vi "SaveTempData3.vi"(2 "temp data":dbl[][][](array[numeric]), 3 "Exp_params":T3={"filename"="201612011532", "ExpFilePath"=path "\\\\10.0.0.7\\takada2/DATA/HBT6/data/Test/201612011532.h5", "File Ref list"=[16777216, 33554432], "sweep_dim"=[4, 2], "sweep_list"=[], "readout_list"=["ADC0", "ADC1"], "Sweep instrument bools"=[[0, 0], [0, 0], [0, 0], [0, 0], [0, 0], [0, 0], [0, 0], [0, 0], [0, 0], [0, 0], [0, 0], [0, 0], [0, 0], [0, 0], [0, 0], [0, 0], [0, 0], [0, 0], [0, 0], [0, 0], [0, 0], [0, 0], [0, 0], [0, 0], [0, 0], [0, 0], [0, 0], [0, 0], [0, 0], [0, 0], [0, 0]], "Read out instrument bools"=[[1, 0]], "Experimental bool list"=[FALSE, TRUE], "Initial move"=[{"Name"="None", "kind"=100, "Value"=0.0}], "FPGA Ref"=refnum, "Inst_parameters"={"ConfigFilePath"=path "\\\\10.0.0.7\\takada2/DATA/HBT6/data/Configs/HBT6_ramp_1.h5", "Inst_list"=["ADC", "AWG", "Freq", "Power", "sus", "rus", "rls", "sls", "suq", "suu", "sur", "suc", "sul", "ruq", "ruu", "rur", "ruc", "rul", "rlq", "rlu", "rlr", "rlc", "rll", "slq", "slu", "slr", "slc", "sll", "tu", "t", "tl", "fast_sequence"], "fast_mode"=[1, 1], "Wait_times"=[1, 1, 1, 1], "Inst_array"=[{"Kind"=0, "Strings"=["ADC", "", "V", "ADC0;ADC1", "V;V", "1.0;1.0"], "uint64s"=[10, 2, 250000, 0, 100, 10106, 1000000, 1, 0, 1], "Doubles"=[1.0], "DAQmx take out list"=[]}, {"Kind"=7, "Strings"=["AWG", "10.0.0.4", "", "C:\\Documents and Settings\\Bauerle\\Mes documents\\Bautze\\FPGA-clean_works_1.13.6_batchtest\\Python\\AWG", "dummy", "SAWnstrig_v4.py"], "uint64s"=[2, 0, 0, 3, 0, 0, 0, 0, 0, 0, 0, 0, 0, 0], "Doubles"=[1200000000.0, 1.0, 0.0, 1.0, 0.0, 1.0, 0.0, 1.0, 0.0, 1.0, 0.0, 1.0, 0.0], "DAQmx take out list"=[]}, {"Kind"=6, "Strings"=["Freq", "0:19", "GHz"], "uint64s"=[1, 0, 0, 0, 2, 0, 0, 0], "Doubles"=[2.0, -30.0, 200.0, 100.0, 0.0, 6.000999927520752, 9.000000318337698e-06, 30.0, -145.0], "DAQmx take out list"=[]}, {"Kind"=6, "Strings"=["Power", "0:19", "GHz"], "uint64s"=[1, 0, 1, 0, 2, 0, 0, 0], "Doubles"=[2.0, -30.0, 200.0, 100.0, 0.0, 6.000999927520752, 9.000000318337698e-06, 30.0, -145.0], "DAQmx take out list"=[]}, {"Kind"=4, "Strings"=["sus", "10.0.0.2", "mV"], "uint64s"=[0, 1], "Doubles"=[1.0, -1.0, 1.0, -1.0, 1.0], "DAQmx take out list"=[]}, {"Kind"=4, "Strings"=["rus", "10.0.0.2", "mV"], "uint64s"=[0, 2], "Doubles"=[1.0, -1.0, 1.0, -1.0, 1.0], "DAQmx take out list"=[]}, {"Kind"=4, "Strings"=["rls", "10.0.0.2", "mV"], "uint64s"=[0, 3], "Doubles"=[1.0, -1.0, 1.0, -1.0, 1.0], "DAQmx take out list"=[]}, {"Kind"=4, "Strings"=["sls", "10.0.0.2", "mV"], "uint64s"=[0, 4], "Doubles"=[1.0, -1.0, 1.0, -1.0, 1.0], "DAQmx take out list"=[]}, {"Kind"=4, "Strings"=["suq", "10.0.0.2", "V"], "uint64s"=[0, 5], "Doubles"=[0.30000001192092896, -2.0, 1.0, -1.0, 1.0], "DAQmx take out list"=[]}, {"Kind"=4, "Strings"=["suu", "10.0.0.2", "V"], "uint64s"=[0, 6], "Doubles"=[0.30000001192092896, -2.0, 1.0, -1.0, 1.0], "DAQmx take out list"=[]}, {"Kind"=4, "Strings"=["sur", "10.0.0.2", "V"], "uint64s"=[0, 7], "Doubles"=[0.30000001192092896, -2.0, 1.0, -1.0, 1.0], "DAQmx take out list"=[]}, {"Kind"=4, "Strings"=["suc", "10.0.0.2", "V"], "uint64s"=[1, 0], "Doubles"=[0.30000001192092896, -2.0, 1.0, -1.0, 1.0], "DAQmx take out list"=[]}, {"Kind"=4, "Strings"=["sul", "10.0.0.2", "V"], "uint64s"=[1, 1], "Doubles"=[0.30000001192092896, -2.0, 1.0, -1.0, 1.0], "DAQmx take out list"=[]}, {"Kind"=4, "Strings"=["ruq", "10.0.0.2", "V"], "uint64s"=[1, 2], "Doubles"=[0.30000001192092896, -2.0, 1.0, -1.0, 1.0], "DAQmx take out list"=[]}, {"Kind"=4, "Strings"=["ruu", "10.0.0.2", "V"], "uint64s"=[1, 3], "Doubles"=[0.30000001192092896, -2.0, 1.0, -1.0, 1.0], "DAQmx take out list"=[]}, {"Kind"=4, "Strings"=["rur", "10.0.0.2", "V"], "uint64s"=[1, 5], "Doubles"=[0.30000001192092896, -2.0, 1.0, -1.0, 1.0], "DAQmx take out list"=[]}, {"Kind"=4, "Strings"=["ruc", "10.0.0.2", "V"], "uint64s"=[1, 6], "Doubles"=[0.30000001192092896, -2.0, 1.0, -1.0, 1.0], "DAQmx take out list"=[]}, {"Kind"=4, "Strings"=["rul", "10.0.0.2", "V"], "uint64s"=[1, 7], "Doubles"=[0.30000001192092896, -2.0, 1.0, -1.0, 1.0], "DAQmx take out list"=[]}, {"Kind"=4, "Strings"=["rlq", "10.0.0.2", "V"], "uint64s"=[2, 0], "Doubles"=[0.30000001192092896, -2.0, 1.0, -1.0, 1.0], "DAQmx take out list"=[]}, {"Kind"=4, "Strings"=["rlu", "10.0.0.2", "V"], "uint64s"=[2, 1], "Doubles"=[0.30000001192092896, -2.0, 1.0, -1.0, 1.0], "DAQmx take out list"=[]}, {"Kind"=4, "Strings"=["rlr", "10.0.0.2", "V"], "uint64s"=[2, 2], "Doubles"=[0.30000001192092896, -2.0, 1.0, -1.0, 1.0], "DAQmx take out list"=[]}, {"Kind"=4, "Strings"=["rlc", "10.0.0.2", "V"], "uint64s"=[2, 3], "Doubles"=[0.30000001192092896, -2.0, 1.0, -1.0, 1.0], "DAQmx take out list"=[]}, {"Kind"=4, "Strings"=["rll", "10.0.0.2", "V"], "uint64s"=[2, 4], "Doubles"=[0.30000001192092896, -2.0, 1.0, -1.0, 1.0], "DAQmx take out list"=[]}, {"Kind"=4, "Strings"=["slq", "10.0.0.2", "V"], "uint64s"=[2, 5], "Doubles"=[0.30000001192092896, -2.0, 1.0, -1.0, 1.0], "DAQmx take out list"=[]}, {"Kind"=4, "Strings"=["slu", "10.0.0.2", "V"], "uint64s"=[2, 6], "Doubles"=[0.30000001192092896, -2.0, 1.0, -1.0, 1.0], "DAQmx take out list"=[]}, {"Kind"=4, "Strings"=["slr", "10.0.0.2", "V"], "uint64s"=[2, 7], "Doubles"=[0.30000001192092896, -2.0, 1.0, -1.0, 1.0], "DAQmx take out list"=[]}, {"Kind"=4, "Strings"=["slc", "10.0.0.2", "V"], "uint64s"=[3, 0], "Doubles"=[0.30000001192092896, -2.0, 1.0, -1.0, 1.0], "DAQmx take out list"=[]}, {"Kind"=4, "Strings"=["sll", "10.0.0.2", "V"], "uint64s"=[3, 1], "Doubles"=[0.30000001192092896, -2.0, 1.0, -1.0, 1.0], "DAQmx take out list"=[]}, {"Kind"=4, "Strings"=["tu", "10.0.0.2", "V"], "uint64s"=[3, 2], "Doubles"=[0.30000001192092896, -2.0, 1.0, -1.0, 1.0], "DAQmx take out list"=[]}, {"Kind"=4, "Strings"=["t", "10.0.0.2", "V"], "uint64s"=[3, 3], "Doubles"=[0.30000001192092896, -2.0, 1.0, -1.0, 1.0], "DAQmx take out list"=[]}, {"Kind"=4, "Strings"=["tl", "10.0.0.2", "V"], "uint64s"=[3, 4], "Doubles"=[0.30000001192092896, -2.0, 1.0, -1.0, 1.0], "DAQmx take out list"=[]}, {"Kind"=9, "Strings"=["fast_sequence", "10.0.0.2", "V"], "uint64s"=[6661, 300, 200, 0, 0, 1, 2, 3, 4, 5, 6, 7, 16, 17, 18, 19, 20, 21, 22, 23, 0], "Doubles"=[0.5, -0.5, -1.0, -1.0], "DAQmx take out list"=[]}]}} {"File Ref list" format="%.0x"}, 4 "count":i32) -> (0 "count out":i32)   [LabVIEW 2013]
uses:
  <vilib>/addons/h5labview2/base/hid_t.ctl
  fpga-bitfile-ref.ctl
  <vilib>/addons/h5labview2/file/H5Fmode.ctl
  <vilib>/addons/h5labview2/base/lib_path.vi
  <vilib>/addons/h5labview2/base/H5Equery.vi
  <vilib>/addons/h5labview2/dataset/H5Dwrite.llb/H5Dwrite.xnode
  <vilib>/addons/h5labview2/dataset/H5D.lvlib
  <vilib>/addons/h5labview2/space/H5S.lvlib
  <vilib>/addons/h5labview2/file/H5F.lvlib
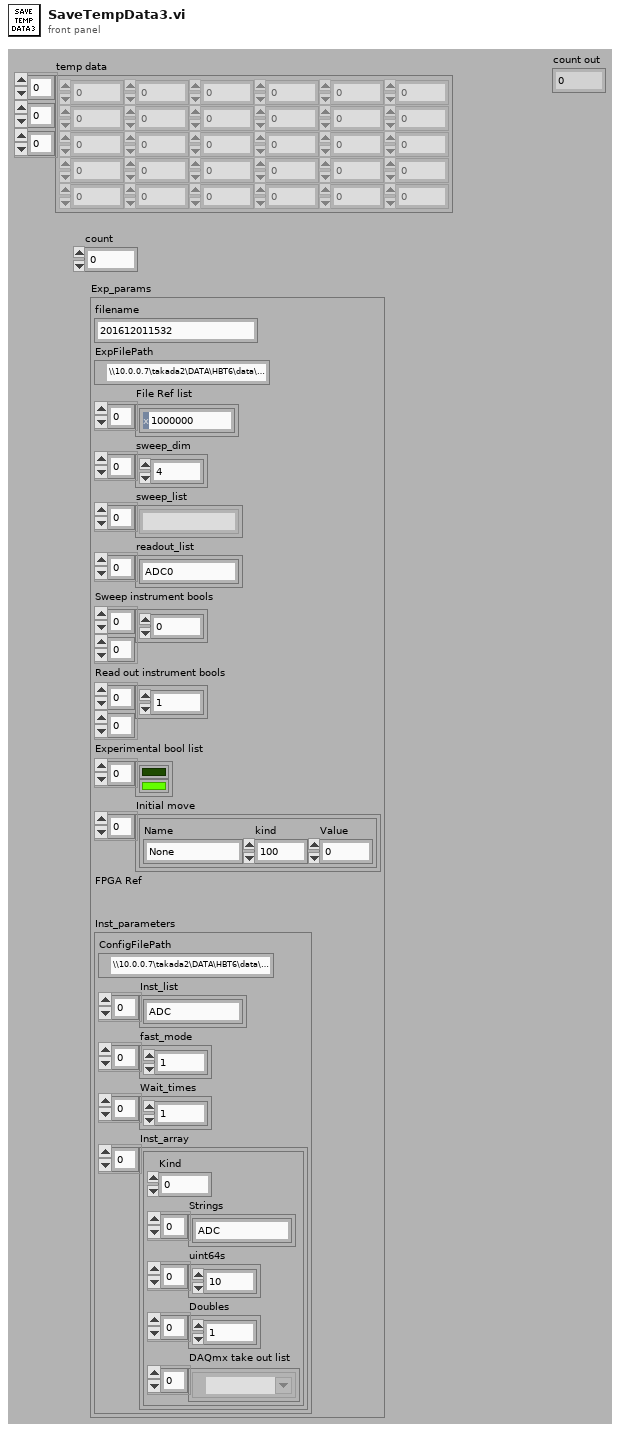
[diagram p1: front panel]
types:
  T1 = typedef "hid_t.ctl" = i32
  T2 = typedef "fpga-bitfile-ref.ctl" = refnum<k20>
  T3 = cluster{"filename":string, "ExpFilePath":path, "File Ref list":T1[], "sweep_dim":u64[], "sweep_list":string[], "readout_list":string[], "Sweep instrument bools":u64[][], "Read out instrument bools":u64[][], "Experimental bool list":bool[], "Initial move":cluster{"Name":string, "kind":u64, "Value":dbl}[], "FPGA Ref":T2, "Inst_parameters":cluster{"ConfigFilePath":path, "Inst_list":string[], "fast_mode":u8[], "Wait_times":u64[], "Inst_array":cluster{"Kind":u16, "Strings":string[], "uint64s":u64[], "Doubles":dbl[], "DAQmx take out list":refnum<k21>[]}[]}}
  T4 = typedef "H5F.lvlib/H5Fmode.ctl" = enum16{"read-only", "read-write", "overwrite", "create new", "open or create"}
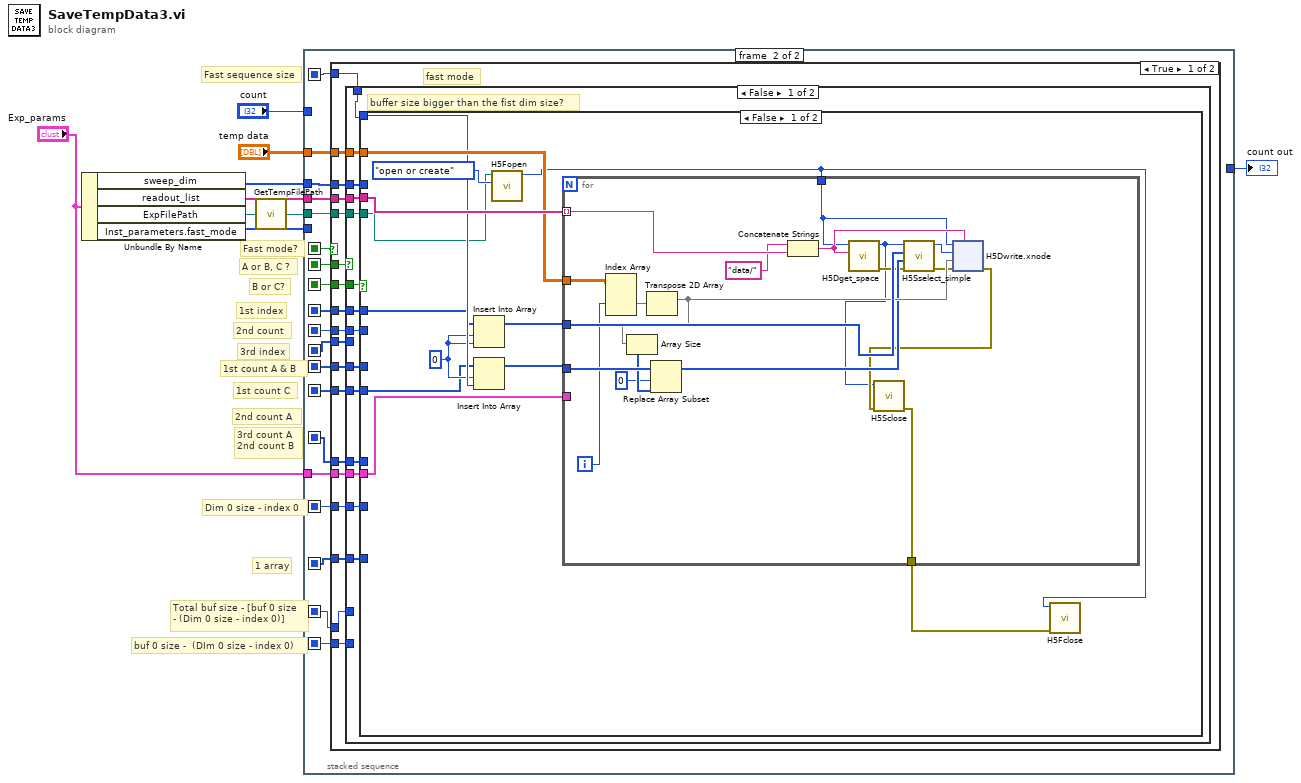
[diagram p0: block diagram]
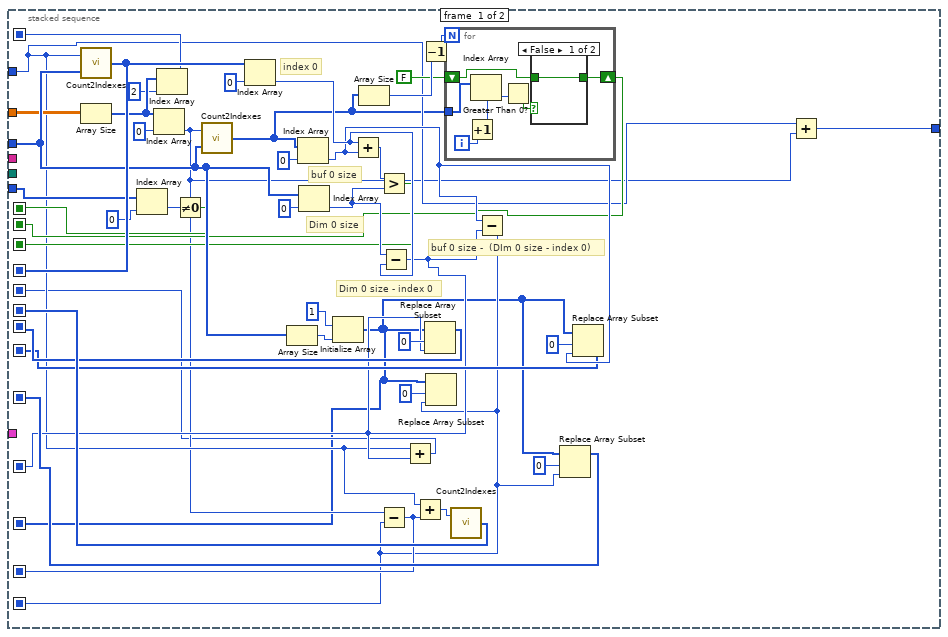
[diagram p2: hidden frame]
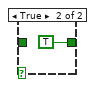
[diagram p3: hidden frame]
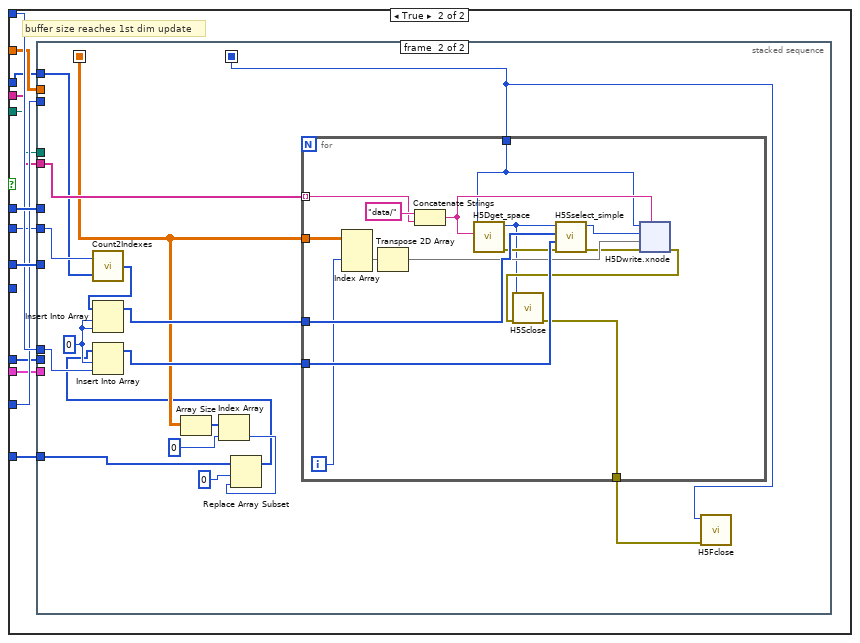
[diagram p4: hidden frame]
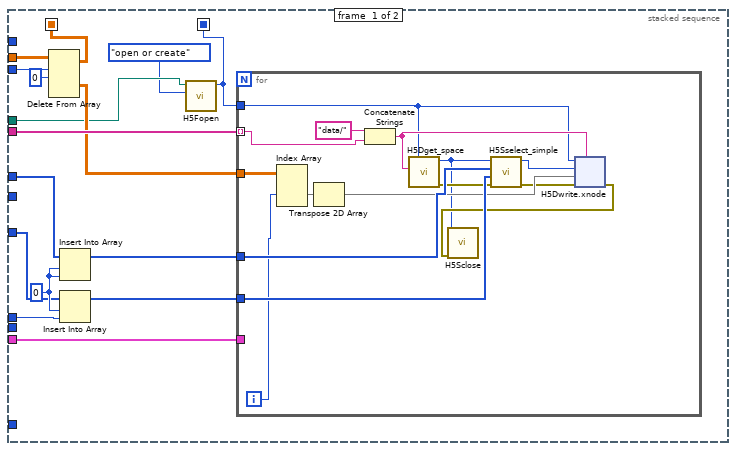
[diagram p5: hidden frame]
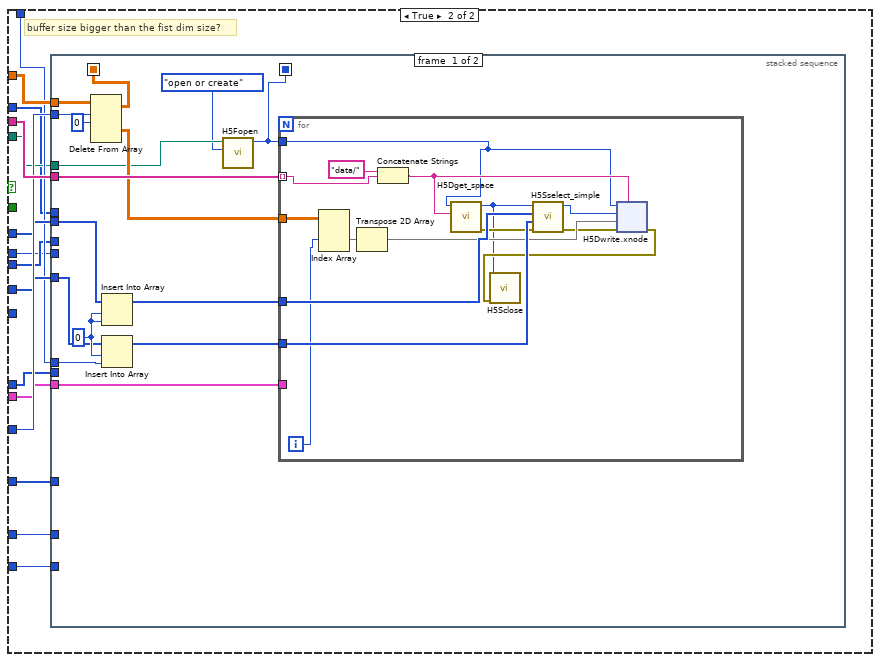
[diagram p6: hidden frame]
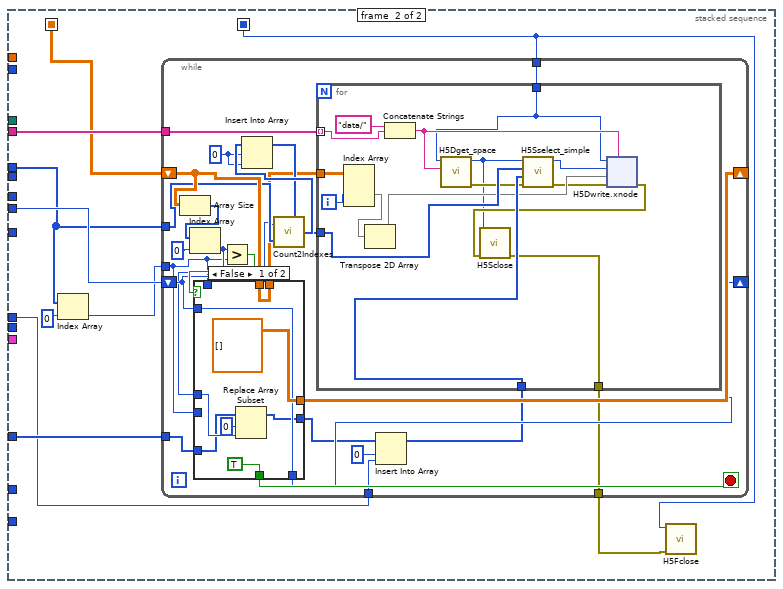
[diagram p7: hidden frame]
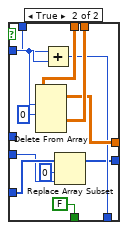
[diagram p8: hidden frame]
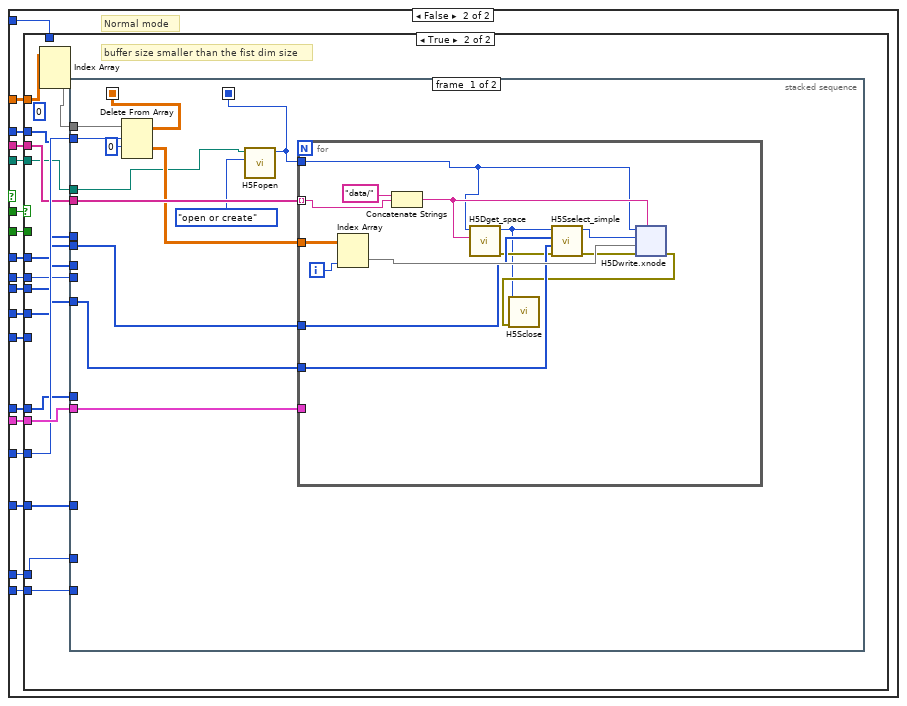
[diagram p9: hidden frame]
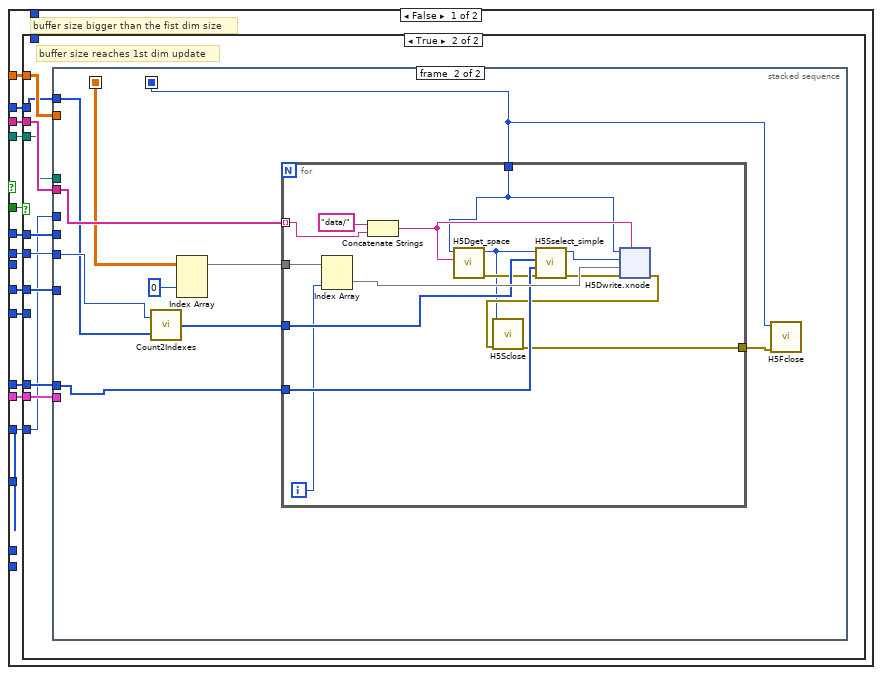
[diagram p10: hidden frame]
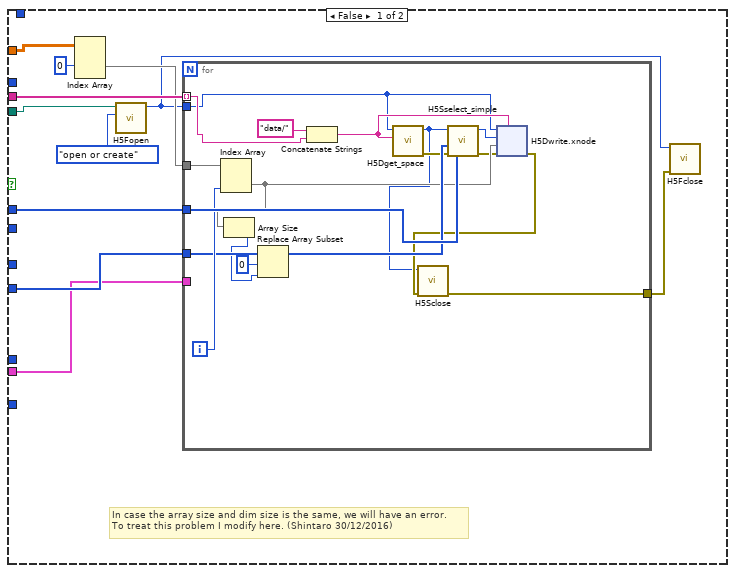
[diagram p11: hidden frame]
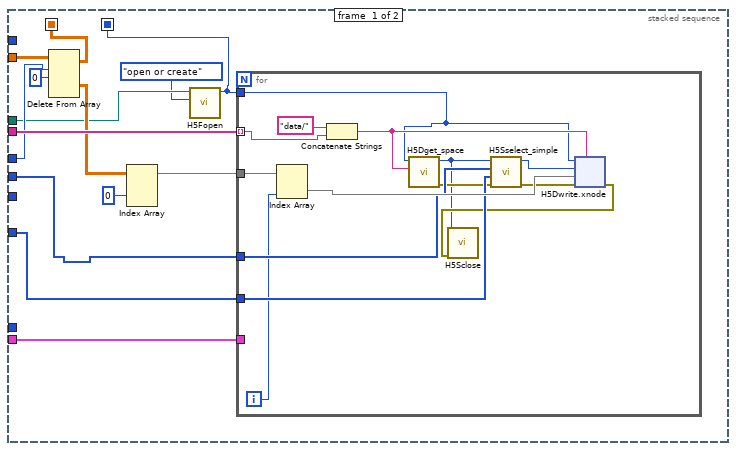
[diagram p12: hidden frame]
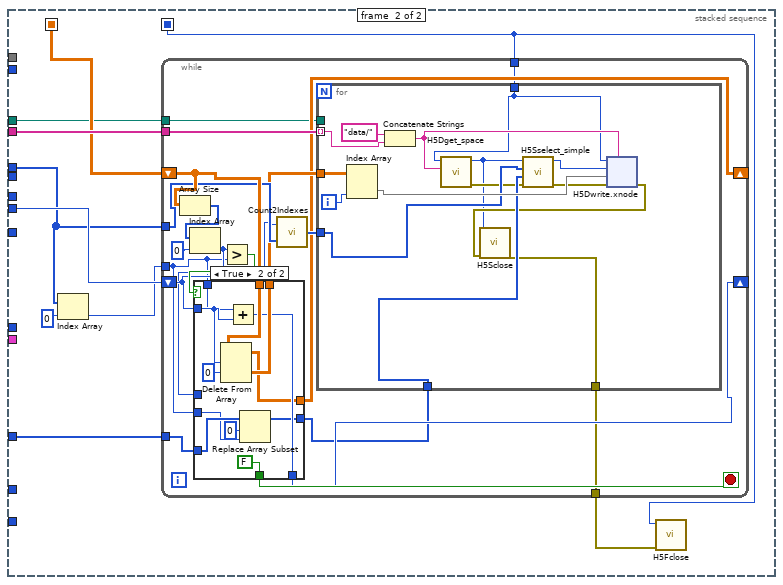
[diagram p13: hidden frame]
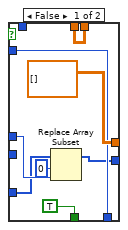
[diagram p14: hidden frame]
diagram:
  # "1 array"
  # "buf 0 size -  (DIm 0 size - index 0)"
  # "Total buf size - [buf 0 size\n- (Dim 0 size - index 0)]"
  # "Dim 0 size - index 0"
  # "Fast sequence size"
  # "B or C?"
  # "A or B, C ?"
  # "Fast mode?"
  # "3rd count A\n2nd count B"
  # "2nd count A"
  # "1st count C"
  # "1st count A & B"
  # "3rd index"
  # "2nd count"
  # "1st index"
  n1 = Unbundle By Name("Exp_params") -> ("sweep_dim"=w7:u64[], "readout_list"=w6:string[], "ExpFilePath"=w2:path, "Inst_parameters.fast_mode"=w5:u8[])
  n2 = call "GetTempFilePath.vi"("ExpFilePath"=w2) -> ("Temp file path"=w1:path)
  n3 = stacked-sequence {
    seq-local: [w48 _] -> [_ w74]
    seq-local: [w11 _] -> [_ w67]
    seq-local: [w36 _] -> [_ w66]
    seq-local: [w35 _] -> [_ w70]
    seq-local: [w32 _] -> [_ w73]
    seq-local: [w29 _] -> [_ w68]
    seq-local: [w22 _] -> [_ w80]
    seq-local: [w26 _] -> [_ w79]
    seq-local: [w27 _] -> [_ w78]
    seq-local: [w19 _] -> [_ w71]
    seq-local: [w18 _] -> [_ w69]
    seq-local: [w14 _] -> [_ w65]
    seq-local: [w13 _] -> [_ w64]
    seq-local: [w10 _] -> [_ w62]
    tunnel: "count" -> [w17 _]
    tunnel: "temp data" -> [w28 w77]
    tunnel: w1 -> [_ w75]
    tunnel: w7 -> [w38 w63]
    tunnel: w6 -> [_ w76]
    tunnel: w5 -> [w25 _]
    tunnel: "Exp_params" -> [_ w72]
    tunnel: [w16 _] -> w3
    frame #0 {
      # "buf 0 size -  (DIm 0 size - index 0)"
      # "Dim 0 size - index 0"
      # "Dim 0 size"
      # "buf 0 size"
      # "index 0"
      n4 = call "Count2Indexes.vi"("sweep_dim"=w38, "Count"=w17) -> ("Indexes"=w48:u64[])
      n5 = Array Size(array=w28) -> (size(s)=w21:i32[])
      n6 = Index Array(array=w25, index=0) -> (element=w23:u8)
      n7 = Index Array(array=w21, index=0) -> (element=w15:i32)
      n8 = Index Array(array=w21, index=2) -> (element=w19:i32)
      n9 = Not Equal To 0?(x=w23) -> (x != 0?=w22:bool)
      n10 = call "Count2Indexes.vi"("sweep_dim"=w38, "Count"=w15) -> ("Indexes"=w12:u64[])
      n11 = Index Array(array=w48, index=0) -> (element=w43:u64)
      n12 = Array Size(array=w38) -> (size(s)=w42:i32)
      n13 = Index Array(array=w12, index=0) -> (element=w33:u64)
      n14 = Index Array(array=w38, index=0) -> (element=w31:u64)
      n15 = Initialize Array(1, w42) -> (w10:i32[])
      n16 = Add(x=w43, y=w33) -> (x+y=w47:u64)
      n17 = Array Size(array=w12) -> (size(s)=w46:i32)
      n18 = Greater?(x=w47, y=w31) -> (0:w27:bool)
      n19 = Subtract(x=w31, y=w43) -> (x-y=w18:u64)
      n20 = Add(x=w17, y=w18) -> (x+y=w11:u64)
      n21 = Decrement(x=w46) -> (x-1=w45:i32)
      n22 = Replace Array Subset(array=w10, new element=w18, index=0) -> (w35:i32[])
      n23 = for {
        N: w45 -> [_]
        tunnel: w12 -> [w59]
        shift-right: [w53] -> w26
        shift-left: FALSE -> [w54]
        i -> [w58]
        n24 = Increment(x=w58) -> (x+1=w57:i32)
        n25 = Index Array(array=w59, index=w57) -> (element=w56:u64)
        n26 = Greater Than 0?(x=w56) -> (x > 0?=w55:bool)
        n27 = case shown="False" w55 {
          tunnel: w54 -> [w60 _]
          tunnel: [w60 TRUE] -> w53
          frame False {
          }
          frame True {
          }
        }
      }
      n28 = Subtract(x=w33, y=w18) -> (x-y=w13:u64)
      n29 = Subtract(x=w15, y=w13) -> (x-y=w14:u64)
      n30 = Add(x=w17, y=w14) -> (x+y=w37:u64)
      n31 = Replace Array Subset(array=w10, new element=w13, index=0) -> ()  [unwired: 1 out]
      n32 = call "Count2Indexes.vi"("Count"=w37) -> ("Indexes"=w36:u64[])  [unwired: 1 in]
      n33 = Replace Array Subset(array=w10, new element=w13, index=0) -> (w29:i32[])
      n34 = Replace Array Subset(array=w10, new element=w33, index=0) -> (w32:i32[])
      n35 = Add(x=w17, y=w15) -> (x+y=w16:i32)
    }
    frame #1 {
      n36 = case shown="True" w80 {
        tunnel: w79 -> [w98 w443]
        tunnel: w78 -> [w97 w442]
        tunnel: w77 -> [w95 w441]
        tunnel: w76 -> [w96 w440]
        tunnel: w75 -> [w94 w439]
        tunnel: w74 -> [w91 w438]
        tunnel: w73 -> [w90 w437]
        tunnel: w72 -> [w93 w436]
        tunnel: w71 -> [w92 w434]
        tunnel: w70 -> [w89 w435]
        tunnel: w69 -> [w88 w431]
        tunnel: w68 -> [w87 w433]
        tunnel: w67 -> [w86 w432]
        tunnel: w66 -> [w85 w426]
        tunnel: w65 -> [w84 w430]
        tunnel: w64 -> [w83 w429]
        tunnel: w63 -> [w82 w428]
        tunnel: w62 -> [w81 w427]
        frame True {
          # "fast mode"
          n37 = case shown="False" w98 {
            tunnel: w97 -> [w112 _]
            tunnel: w96 -> [w111 w288]
            tunnel: w95 -> [w110 w289]
            tunnel: w94 -> [w109 w280]
            tunnel: w93 -> [w108 w283]
            tunnel: w92 -> [w107 w284]
            tunnel: w91 -> [w106 w286]
            tunnel: w90 -> [w105 _]
            tunnel: w89 -> [w104 w285]
            tunnel: w88 -> [w103 w287]
            tunnel: w87 -> [w102 w281]
            tunnel: w86 -> [w101 w279]
            tunnel: w85 -> [_ w282]
            tunnel: w84 -> [_ w278]
            tunnel: w83 -> [_ w277]
            tunnel: w82 -> [w100 w276]
            tunnel: w81 -> [w99 w275]
            frame False {
              # "buffer size bigger than the fist dim size?"
              n38 = case shown="False" w112 {
                tunnel: w111 -> [w125 w169]
                tunnel: w110 -> [w124 w171]
                tunnel: w109 -> [w115 w168]
                tunnel: w108 -> [w123 w167]
                tunnel: w107 -> [w122 w172]
                tunnel: w106 -> [w120 w173]
                tunnel: w105 -> [w119 _]
                tunnel: w104 -> [_ w174]
                tunnel: w103 -> [_ w170]
                tunnel: w102 -> [_ w166]
                tunnel: w101 -> [_ w165]
                tunnel: w100 -> [_ w164]
                tunnel: w99 -> [_ w163]
                frame False {
                  w121 = 0
                  n39 = Insert Into Array(array=w120, index=w121, new element=w121) -> (w118:u64[])
                  n40 = Insert Into Array(array=w119, index=w121, new element=w122) -> (w117:i32[])
                  n41 = call <vilib>:"H5Fopen.vi"("mode (read-only)"=H5Fmode."open or create" ("mode"), "path"=w115) -> ("ref out"=w113:T1)  [unwired: 8 in, 1 out]
                  n42 = for {
                    tunnel: w118 -> [w144]
                    tunnel: w125 -> [w143] mode=indexing
                    tunnel: w124 -> [w142]
                    tunnel: w117 -> [w140]
                    tunnel: w123 -> [_]
                    tunnel: w113 -> [w127]
                    tunnel: [w126] -> w114
                    i -> [w139]
                    n43 = Index Array(array=w142, index (dim 1)=w139) -> (element=w141:dbl[][])  [unwired: 2 in]
                    n44 = Transpose 2D Array(2D array=w141) -> (transposed array=w138:dbl[][])
                    n45 = Array Size(array=w138) -> (size(s)=w136:i32[])
                    n46 = Replace Array Subset(array=w140, new element=w136, index=0) -> (w137:i32[])
                    n47 = Concatenate Strings("data/", w143) -> (w129:string)
                    n48 = call <vilib>:"H5Dget_space.vi"("obj (.)"=w129, "ref in"=w127) -> ("error out"=w134:errorcluster, "space out"=w130:T1)  [unwired: 8 in]
                    n49 = call <vilib>:"H5Sselect_simple.vi"("error in (no error)"=w134, "count"=w137, "start"=w144, "space in"=w130) -> ("error out"=w133:errorcluster, "space out"=w132:T1)  [unwired: 6 in]
                    n50 = xnode "H5Dwrite.xnode"("dataset name"=w129, "error in (no error)"=w133, "data"=w138, "file space"=w132, "ref in"=w127) -> ("error out"=w131:errorcluster)  [unwired: 2 in, 2 out]
                    n51 = call <vilib>:"H5Sclose.vi"("error in (no error)"=w131, "space in"=w130) -> ("error out"=w126:errorcluster)  [unwired: 9 in]
                  }
                  n52 = call <vilib>:"H5Fclose.vi"("error in (no error)"=w114, "ref"=w113) -> ()  [unwired: 9 in, 1 out]
                }
                frame True {
                  # "buffer size reaches 1st dim update"
                  n53 = stacked-sequence {
                    seq-local: [w183 _] -> [_ w232]
                    seq-local: [w175 _] -> [_ w224]
                    tunnel: w174 -> [w189 _]
                    tunnel: w173 -> [w188 _]
                    tunnel: w172 -> [w187 w238]
                    tunnel: w171 -> [w186 _]
                    tunnel: w170 -> [w185 _]
                    tunnel: w169 -> [w182 w240]
                    tunnel: w168 -> [w177 _]
                    tunnel: w167 -> [w178 _]
                    tunnel: w166 -> [_ _]
                    tunnel: w165 -> [_ w235]
                    tunnel: w164 -> [_ w233]
                    tunnel: w163 -> [_ w229]
                    frame #0 {
                      w190 = 0
                      n54 = Delete From Array(array=w186, length=w185, index (dim 0)=0) -> (deleted portion=w181:dbl[][][], array with subset deleted=w183:dbl[][][])  [unwired: 2 in]
                      n55 = Insert Into Array(array=w188, index=w190, new element=w190) -> (w179:u64[])
                      n56 = Insert Into Array(array=w189, index=w190, new element=w187) -> (w180:i32[])
                      n57 = call <vilib>:"H5Fopen.vi"("mode (read-only)"=H5Fmode."open or create" ("mode"), "path"=w177) -> ("ref out"=w175:T1)  [unwired: 8 in, 1 out]
                      n58 = for {
                        tunnel: w182 -> [w193] mode=indexing
                        tunnel: w181 -> [w205]
                        tunnel: w180 -> [w203]
                        tunnel: w179 -> [w202]
                        tunnel: w178 -> [_]
                        tunnel: w175 -> [w191]
                        i -> [w201]
                        n59 = Index Array(array=w205, index (dim 1)=w201) -> (element=w204:dbl[][])  [unwired: 2 in]
                        n60 = Transpose 2D Array(2D array=w204) -> (transposed array=w200:dbl[][])
                        n61 = Concatenate Strings("data/", w193) -> (w192:string)
                        n62 = call <vilib>:"H5Dget_space.vi"("obj (.)"=w192, "ref in"=w191) -> ("error out"=w199:errorcluster, "space out"=w195:T1)  [unwired: 8 in]
                        n63 = call <vilib>:"H5Sselect_simple.vi"("error in (no error)"=w199, "count"=w203, "start"=w202, "space in"=w195) -> ("error out"=w198:errorcluster, "space out"=w197:T1)  [unwired: 6 in]
                        n64 = xnode "H5Dwrite.xnode"("dataset name"=w192, "error in (no error)"=w198, "data"=w200, "file space"=w197, "ref in"=w191) -> ("error out"=w196:errorcluster)  [unwired: 2 in, 2 out]
                        n65 = call <vilib>:"H5Sclose.vi"("error in (no error)"=w196, "space in"=w195) -> ()  [unwired: 9 in, 1 out]
                      }
                    }
                    frame #1 {
                      w239 = 0
                      n66 = call "Count2Indexes.vi"("sweep_dim"=w233, "Count"=w235) -> ("Indexes"=w234:u64[])
                      n67 = Insert Into Array(array=w234, index=w239, new element=w239) -> (w236:u64[])
                      n68 = Array Size(array=w232) -> (size(s)=w231:i32[])
                      n69 = Index Array(array=w231, index=0) -> (element=w228:i32)
                      n70 = Replace Array Subset(array=w229, new element=w228, index=0) -> (w226:i32[])
                      n71 = Insert Into Array(array=w226, index=w239, new element=w238) -> (w237:i32[])
                      n72 = for {
                        tunnel: w240 -> [w244] mode=indexing
                        tunnel: w232 -> [w256]
                        tunnel: w237 -> [w254]
                        tunnel: w236 -> [w253]
                        tunnel: w224 -> [w242]
                        tunnel: [w241] -> w225
                        i -> [w252]
                        n73 = Index Array(array=w256, index (dim 1)=w252) -> (element=w255:dbl[][])  [unwired: 2 in]
                        n74 = Transpose 2D Array(2D array=w255) -> (transposed array=w251:dbl[][])
                        n75 = Concatenate Strings("data/", w244) -> (w243:string)
                        n76 = call <vilib>:"H5Dget_space.vi"("obj (.)"=w243, "ref in"=w242) -> ("error out"=w250:errorcluster, "space out"=w246:T1)  [unwired: 8 in]
                        n77 = call <vilib>:"H5Sselect_simple.vi"("error in (no error)"=w250, "count"=w254, "start"=w253, "space in"=w246) -> ("error out"=w249:errorcluster, "space out"=w248:T1)  [unwired: 6 in]
                        n78 = xnode "H5Dwrite.xnode"("dataset name"=w243, "error in (no error)"=w249, "data"=w251, "file space"=w248, "ref in"=w242) -> ("error out"=w247:errorcluster)  [unwired: 2 in, 2 out]
                        n79 = call <vilib>:"H5Sclose.vi"("error in (no error)"=w247, "space in"=w246) -> ("error out"=w241:errorcluster)  [unwired: 9 in]
                      }
                      n80 = call <vilib>:"H5Fclose.vi"("error in (no error)"=w225, "ref"=w224) -> ()  [unwired: 9 in, 1 out]
                    }
                  }
                }
              }
            }
            frame True {
              # "buffer size bigger than the fist dim size?"
              n81 = stacked-sequence {
                seq-local: [w298 _] -> [_ w341]
                seq-local: [w290 _] -> [_ w339]
                tunnel: w285 -> [w304 _]
                tunnel: w286 -> [w303 _]
                tunnel: w284 -> [w302 w342]
                tunnel: w289 -> [w301 _]
                tunnel: w287 -> [w300 _]
                tunnel: w288 -> [w297 w348]
                tunnel: w280 -> [w292 _]
                tunnel: w283 -> [w294 _]
                tunnel: w281 -> [_ _]
                tunnel: w282 -> [_ _]
                tunnel: w279 -> [_ w347]
                tunnel: w278 -> [_ _]
                tunnel: w277 -> [_ _]
                tunnel: w276 -> [_ w346]
                tunnel: w275 -> [_ w343]
                frame #0 {
                  w305 = 0
                  n82 = Delete From Array(array=w301, length=w300, index (dim 0)=0) -> (deleted portion=w296:dbl[][][], array with subset deleted=w298:dbl[][][])  [unwired: 2 in]
                  n83 = Insert Into Array(array=w303, index=w305, new element=w305) -> (w295:u64[])
                  n84 = Insert Into Array(array=w304, index=w305, new element=w302) -> (w293:i32[])
                  n85 = call <vilib>:"H5Fopen.vi"("mode (read-only)"=H5Fmode."open or create" ("mode"), "path"=w292) -> ("ref out"=w290:T1)  [unwired: 8 in, 1 out]
                  n86 = for {
                    tunnel: w297 -> [w308] mode=indexing
                    tunnel: w296 -> [w320]
                    tunnel: w293 -> [w318]
                    tunnel: w295 -> [w317]
                    tunnel: w294 -> [_]
                    tunnel: w290 -> [w306]
                    i -> [w316]
                    n87 = Index Array(array=w320, index (dim 1)=w316) -> (element=w319:dbl[][])  [unwired: 2 in]
                    n88 = Transpose 2D Array(2D array=w319) -> (transposed array=w315:dbl[][])
                    n89 = Concatenate Strings("data/", w308) -> (w307:string)
                    n90 = call <vilib>:"H5Dget_space.vi"("obj (.)"=w307, "ref in"=w306) -> ("error out"=w314:errorcluster, "space out"=w310:T1)  [unwired: 8 in]
                    n91 = call <vilib>:"H5Sselect_simple.vi"("error in (no error)"=w314, "count"=w318, "start"=w317, "space in"=w310) -> ("error out"=w313:errorcluster, "space out"=w312:T1)  [unwired: 6 in]
                    n92 = xnode "H5Dwrite.xnode"("dataset name"=w307, "error in (no error)"=w313, "data"=w315, "file space"=w312, "ref in"=w306) -> ("error out"=w311:errorcluster)  [unwired: 2 in, 2 out]
                    n93 = call <vilib>:"H5Sclose.vi"("error in (no error)"=w311, "space in"=w310) -> ()  [unwired: 9 in, 1 out]
                  }
                }
                frame #1 {
                  n94 = Index Array(array=w346, index=0) -> (element=w344:u64)
                  n95 = while {
                    tunnel: w348 -> [w371]
                    shift-right: [w365] -> _
                    shift-left: w341 -> [w367]
                    tunnel: w346 -> [w363]
                    shift-right: [w364] -> _
                    shift-left: w347 -> [w362]
                    tunnel: w344 -> [w356]
                    tunnel: w343 -> [w355]
                    tunnel: w342 -> [w352]
                    tunnel: w339 -> [w350]
                    tunnel: [w349] -> w340
                    stop <- w366 stop-if-true
                    w360 = 0
                    n96 = Array Size(array=w367) -> (size(s)=w370:i32[])
                    n97 = Index Array(array=w370, index=0) -> (element=w357:i32)
                    n98 = Greater?(x=w357, y=w356) -> (0:w368:bool)
                    n99 = case shown="False" w368 {
                      tunnel: w362 -> [w376 w391]
                      tunnel: w356 -> [_ w387]
                      tunnel: w367 -> [w378 w390]
                      tunnel: [w378 w389] -> w358
                      tunnel: [TRUE FALSE] -> w366
                      tunnel: [dbl[][][] [] w385] -> w365
                      tunnel: [w376 w384] -> w364
                      tunnel: w357 -> [w373 _]
                      tunnel: w356 -> [_ w382]
                      tunnel: w355 -> [w372 w383]
                      tunnel: [w374 w380] -> w354
                      frame False {
                        n100 = Replace Array Subset(array=w372, new element=w373, index=0) -> (w374:i32[])
                      }
                      frame True {
                        n101 = Delete From Array(array=w390, length=w387, index (dim 0)=0) -> (deleted portion=w389:dbl[][][], array with subset deleted=w385:dbl[][][])  [unwired: 2 in]
                        n102 = Add(x=w387, y=w391) -> (x+y=w384:u64)
                        n103 = Replace Array Subset(array=w383, new element=w382, index=0) -> (w380:i32[])
                      }
                    }
                    n104 = call "Count2Indexes.vi"("sweep_dim"=w363, "Count"=w362) -> ("Indexes"=w361:u64[])
                    n105 = Insert Into Array(array=w361, index=w360, new element=w360) -> (w359:u64[])
                    n106 = Insert Into Array(array=w354, index=0, new element=w352) -> (w351:i32[])
                    n107 = for {
                      tunnel: w371 -> [w395] mode=indexing
                      tunnel: w358 -> [w407]
                      tunnel: w359 -> [w406]
                      tunnel: w351 -> [w405]
                      tunnel: w350 -> [w393]
                      tunnel: [w392] -> w349
                      i -> [w404]
                      n108 = Index Array(array=w407, index (dim 1)=w404) -> (element=w403:dbl[][])  [unwired: 2 in]
                      n109 = Transpose 2D Array(2D array=w403) -> (transposed array=w402:dbl[][])
                      n110 = Concatenate Strings("data/", w395) -> (w394:string)
                      n111 = call <vilib>:"H5Dget_space.vi"("obj (.)"=w394, "ref in"=w393) -> ("error out"=w401:errorcluster, "space out"=w397:T1)  [unwired: 8 in]
                      n112 = call <vilib>:"H5Sselect_simple.vi"("error in (no error)"=w401, "count"=w405, "start"=w406, "space in"=w397) -> ("error out"=w400:errorcluster, "space out"=w399:T1)  [unwired: 6 in]
                      n113 = xnode "H5Dwrite.xnode"("dataset name"=w394, "error in (no error)"=w400, "data"=w402, "file space"=w399, "ref in"=w393) -> ("error out"=w398:errorcluster)  [unwired: 2 in, 2 out]
                      n114 = call <vilib>:"H5Sclose.vi"("error in (no error)"=w398, "space in"=w397) -> ("error out"=w392:errorcluster)  [unwired: 9 in]
                    }
                  }
                  n115 = call <vilib>:"H5Fclose.vi"("error in (no error)"=w340, "ref"=w339) -> ()  [unwired: 9 in, 1 out]
                }
              }
            }
          }
        }
        frame False {
          # "Normal mode"
          n116 = case shown="True" w443 {
            tunnel: w442 -> [w456 _]
            tunnel: w441 -> [w455 w605]
            tunnel: w440 -> [w454 w616]
            tunnel: w439 -> [w453 w615]
            tunnel: w438 -> [w452 w614]
            tunnel: w437 -> [w451 _]
            tunnel: w436 -> [w450 w618]
            tunnel: w435 -> [w449 w613]
            tunnel: w434 -> [w448 _]
            tunnel: w433 -> [w447 w606]
            tunnel: w432 -> [w446 w609]
            tunnel: w431 -> [w445 w617]
            tunnel: w430 -> [_ w612]
            tunnel: w429 -> [_ w611]
            tunnel: w428 -> [w444 w610]
            tunnel: w427 -> [_ w608]
            tunnel: w426 -> [_ w607]
            frame False {
              # "buffer size bigger than the fist dim size"
              n117 = case shown="True" w456 {
                tunnel: w455 -> [w465 w513]
                tunnel: w454 -> [w466 w512]
                tunnel: w453 -> [w460 w511]
                tunnel: w452 -> [w467 w510]
                tunnel: w451 -> [w462 _]
                tunnel: w450 -> [w461 w508]
                tunnel: w449 -> [_ w509]
                tunnel: w448 -> [_ _]
                tunnel: w447 -> [_ w507]
                tunnel: w446 -> [_ w506]
                tunnel: w445 -> [_ w505]
                tunnel: w444 -> [_ w504]
                frame False {
                  # "In case the array size and dim size is the same, we will have an error.\nTo treat this problem I modify here. (Shintaro 30/12/2016)"
                  n118 = Index Array(array=w465, index (dim 1)=0) -> (element=w463:dbl[][])  [unwired: 2 in]
                  n119 = call <vilib>:"H5Fopen.vi"("mode (read-only)"=H5Fmode."open or create" ("mode"), "path"=w460) -> ("ref out"=w457:T1)  [unwired: 8 in, 1 out]
                  n120 = for {
                    tunnel: w467 -> [w485]
                    tunnel: w466 -> [w470] mode=indexing
                    tunnel: w463 -> [w484]
                    tunnel: w462 -> [w482]
                    tunnel: w461 -> [_]
                    tunnel: w457 -> [w469]
                    tunnel: [w468] -> w458
                    i -> [w483]
                    n121 = Index Array(array=w484, index (col)=w483) -> (element=w479:dbl[])  [unwired: 1 in]
                    n122 = Array Size(array=w479) -> (size(s)=w478:i32)
                    n123 = Replace Array Subset(array=w482, new element=w478, index=0) -> (w481:i32[])
                    n124 = Concatenate Strings("data/", w470) -> (w471:string)
                    n125 = call <vilib>:"H5Dget_space.vi"("obj (.)"=w471, "ref in"=w469) -> ("error out"=w477:errorcluster, "space out"=w473:T1)  [unwired: 8 in]
                    n126 = call <vilib>:"H5Sselect_simple.vi"("error in (no error)"=w477, "count"=w481, "start"=w485, "space in"=w473) -> ("error out"=w476:errorcluster, "space out"=w475:T1)  [unwired: 6 in]
                    n127 = xnode "H5Dwrite.xnode"("dataset name"=w471, "error in (no error)"=w476, "data"=w479, "file space"=w475, "ref in"=w469) -> ("error out"=w474:errorcluster)  [unwired: 2 in, 2 out]
                    n128 = call <vilib>:"H5Sclose.vi"("error in (no error)"=w474, "space in"=w473) -> ("error out"=w468:errorcluster)  [unwired: 9 in]
                  }
                  n129 = call <vilib>:"H5Fclose.vi"("error in (no error)"=w458, "ref"=w457) -> ()  [unwired: 9 in, 1 out]
                }
                frame True {
                  # "buffer size reaches 1st dim update"
                  n130 = stacked-sequence {
                    seq-local: [w525 _] -> [_ w568]
                    seq-local: [w514 _] -> [_ w560]
                    tunnel: w509 -> [w517 _]
                    tunnel: w510 -> [w518 _]
                    tunnel: w513 -> [w527 _]
                    tunnel: w512 -> [w524 w569]
                    tunnel: w511 -> [w516 _]
                    tunnel: w508 -> [w522 _]
                    tunnel: w507 -> [_ w567]
                    tunnel: w506 -> [_ w563]
                    tunnel: w505 -> [w521 _]
                    tunnel: w504 -> [_ w562]
                    frame #0 {
                      n131 = Delete From Array(array=w527, length=w521, index (dim 0)=0) -> (deleted portion=w523:dbl[][][], array with subset deleted=w525:dbl[][][])  [unwired: 2 in]
                      n132 = Index Array(array=w523, index (dim 1)=0) -> (element=w520:dbl[][])  [unwired: 2 in]
                      n133 = call <vilib>:"H5Fopen.vi"("mode (read-only)"=H5Fmode."open or create" ("mode"), "path"=w516) -> ("ref out"=w514:T1)  [unwired: 8 in, 1 out]
                      n134 = for {
                        tunnel: w524 -> [w529] mode=indexing
                        tunnel: w520 -> [w541]
                        tunnel: w517 -> [w539]
                        tunnel: w518 -> [w538]
                        tunnel: w522 -> [_]
                        tunnel: w514 -> [w528]
                        i -> [w537]
                        n135 = Index Array(array=w541, index (col)=w537) -> (element=w540:dbl[])  [unwired: 1 in]
                        n136 = Concatenate Strings("data/", w529) -> (w530:string)
                        n137 = call <vilib>:"H5Dget_space.vi"("obj (.)"=w530, "ref in"=w528) -> ("error out"=w536:errorcluster, "space out"=w532:T1)  [unwired: 8 in]
                        n138 = call <vilib>:"H5Sselect_simple.vi"("error in (no error)"=w536, "count"=w539, "start"=w538, "space in"=w532) -> ("error out"=w535:errorcluster, "space out"=w534:T1)  [unwired: 6 in]
                        n139 = xnode "H5Dwrite.xnode"("dataset name"=w530, "error in (no error)"=w535, "data"=w540, "file space"=w534, "ref in"=w528) -> ("error out"=w533:errorcluster)  [unwired: 2 in, 2 out]
                        n140 = call <vilib>:"H5Sclose.vi"("error in (no error)"=w533, "space in"=w532) -> ()  [unwired: 9 in, 1 out]
                      }
                    }
                    frame #1 {
                      n141 = call "Count2Indexes.vi"("sweep_dim"=w562, "Count"=w563) -> ("Indexes"=w564:u64[])
                      n142 = Index Array(array=w568, index (dim 1)=0) -> (element=w566:dbl[][])  [unwired: 2 in]
                      n143 = for {
                        tunnel: w569 -> [w574] mode=indexing
                        tunnel: w566 -> [w584]
                        tunnel: w567 -> [w582]
                        tunnel: w564 -> [w581]
                        tunnel: w560 -> [w571]
                        tunnel: [w570] -> w561
                        i -> [w580]
                        n144 = Index Array(array=w584, index (col)=w580) -> (element=w583:dbl[])  [unwired: 1 in]
                        n145 = Concatenate Strings("data/", w574) -> (w573:string)
                        n146 = call <vilib>:"H5Dget_space.vi"("obj (.)"=w573, "ref in"=w571) -> ("error out"=w579:errorcluster, "space out"=w575:T1)  [unwired: 8 in]
                        n147 = call <vilib>:"H5Sselect_simple.vi"("error in (no error)"=w579, "count"=w582, "start"=w581, "space in"=w575) -> ("error out"=w578:errorcluster, "space out"=w577:T1)  [unwired: 6 in]
                        n148 = xnode "H5Dwrite.xnode"("dataset name"=w573, "error in (no error)"=w578, "data"=w583, "file space"=w577, "ref in"=w571) -> ("error out"=w576:errorcluster)  [unwired: 2 in, 2 out]
                        n149 = call <vilib>:"H5Sclose.vi"("error in (no error)"=w576, "space in"=w575) -> ("error out"=w570:errorcluster)  [unwired: 9 in]
                      }
                      n150 = call <vilib>:"H5Fclose.vi"("error in (no error)"=w561, "ref"=w560) -> ()  [unwired: 9 in, 1 out]
                    }
                  }
                }
              }
            }
            frame True {
              # "buffer size smaller than the fist dim size"
              n151 = Index Array(array=w605, index (dim 1)=0) -> (element=w603:dbl[][])  [unwired: 2 in]
              n152 = stacked-sequence {
                seq-local: [w627 _] -> [_ w666]
                seq-local: [w619 _] -> [_ w663]
                tunnel: w613 -> [w623 _]
                tunnel: w614 -> [w622 _]
                tunnel: w603 -> [w630 _]
                tunnel: w617 -> [w629 _]
                tunnel: w616 -> [w626 w672]
                tunnel: w615 -> [w620 w665]
                tunnel: w618 -> [w624 _]
                tunnel: w606 -> [_ _]
                tunnel: w607 -> [_ _]
                tunnel: w609 -> [_ w671]
                tunnel: w612 -> [_ _]
                tunnel: w611 -> [_ _]
                tunnel: w610 -> [_ w670]
                tunnel: w608 -> [_ w667]
                frame #0 {
                  n153 = Delete From Array(array=w630, length=w629, index (row)=0) -> (deleted portion=w625:dbl[][], array with subset deleted=w627:dbl[][])  [unwired: 1 in]
                  n154 = call <vilib>:"H5Fopen.vi"("mode (read-only)"=H5Fmode."open or create" ("mode"), "path"=w620) -> ("ref out"=w619:T1)  [unwired: 8 in, 1 out]
                  n155 = for {
                    tunnel: w626 -> [w632] mode=indexing
                    tunnel: w625 -> [w644]
                    tunnel: w623 -> [w642]
                    tunnel: w622 -> [w641]
                    tunnel: w624 -> [_]
                    tunnel: w619 -> [w631]
                    i -> [w640]
                    n156 = Index Array(array=w644, index (col)=w640) -> (element=w643:dbl[])  [unwired: 1 in]
                    n157 = Concatenate Strings("data/", w632) -> (w633:string)
                    n158 = call <vilib>:"H5Dget_space.vi"("obj (.)"=w633, "ref in"=w631) -> ("error out"=w639:errorcluster, "space out"=w635:T1)  [unwired: 8 in]
                    n159 = call <vilib>:"H5Sselect_simple.vi"("error in (no error)"=w639, "count"=w642, "start"=w641, "space in"=w635) -> ("error out"=w638:errorcluster, "space out"=w637:T1)  [unwired: 6 in]
                    n160 = xnode "H5Dwrite.xnode"("dataset name"=w633, "error in (no error)"=w638, "data"=w643, "file space"=w637, "ref in"=w631) -> ("error out"=w636:errorcluster)  [unwired: 2 in, 2 out]
                    n161 = call <vilib>:"H5Sclose.vi"("error in (no error)"=w636, "space in"=w635) -> ()  [unwired: 9 in, 1 out]
                  }
                }
                frame #1 {
                  n162 = Index Array(array=w670, index=0) -> (element=w668:u64)
                  n163 = while {
                    tunnel: w672 -> [w691]
                    shift-right: [w676] -> _
                    shift-left: w666 -> [w687]
                    tunnel: w670 -> [w684]
                    shift-right: [w685] -> _
                    shift-left: w671 -> [w683]
                    tunnel: w668 -> [w680]
                    tunnel: w667 -> [w679]
                    tunnel: w665 -> [w675]
                    tunnel: w663 -> [w674]
                    tunnel: [w673] -> w664
                    stop <- w686 stop-if-true
                    n164 = Array Size(array=w687) -> (size(s)=w690:i32[])
                    n165 = Index Array(array=w690, index=0) -> (element=w681:i32)
                    n166 = Greater?(x=w681, y=w680) -> (0:w688:bool)
                    n167 = case shown="True" w688 {
                      tunnel: w683 -> [w696 w711]
                      tunnel: w680 -> [_ w707]
                      tunnel: w687 -> [w698 w710]
                      tunnel: [w698 w709] -> w682
                      tunnel: [TRUE FALSE] -> w686
                      tunnel: [dbl[][] [] w700] -> w676
                      tunnel: [w696 w705] -> w685
                      tunnel: w681 -> [w693 _]
                      tunnel: w680 -> [_ w703]
                      tunnel: w679 -> [w692 w704]
                      tunnel: [w694 w701] -> w678
                      frame False {
                        n168 = Replace Array Subset(array=w692, new element=w693, index=0) -> (w694:i32[])
                      }
                      frame True {
                        n169 = Delete From Array(array=w710, length=w707, index (row)=0) -> (deleted portion=w709:dbl[][], array with subset deleted=w700:dbl[][])  [unwired: 1 in]
                        n170 = Add(x=w707, y=w711) -> (x+y=w705:u64)
                        n171 = Replace Array Subset(array=w704, new element=w703, index=0) -> (w701:i32[])
                      }
                    }
                    n172 = call "Count2Indexes.vi"("sweep_dim"=w684, "Count"=w683) -> ("Indexes"=w677:u64[])
                    n173 = for {
                      tunnel: w691 -> [w715] mode=indexing
                      tunnel: w682 -> [w726]
                      tunnel: w677 -> [w723]
                      tunnel: w678 -> [w724]
                      tunnel: w675 -> [_]
                      tunnel: w674 -> [w713]
                      tunnel: [w712] -> w673
                      i -> [w722]
                      n174 = Index Array(array=w726, index (col)=w722) -> (element=w725:dbl[])  [unwired: 1 in]
                      n175 = Concatenate Strings("data/", w715) -> (w714:string)
                      n176 = call <vilib>:"H5Dget_space.vi"("obj (.)"=w714, "ref in"=w713) -> ("error out"=w721:errorcluster, "space out"=w717:T1)  [unwired: 8 in]
                      n177 = call <vilib>:"H5Sselect_simple.vi"("error in (no error)"=w721, "count"=w724, "start"=w723, "space in"=w717) -> ("error out"=w720:errorcluster, "space out"=w719:T1)  [unwired: 6 in]
                      n178 = xnode "H5Dwrite.xnode"("dataset name"=w714, "error in (no error)"=w720, "data"=w725, "file space"=w719, "ref in"=w713) -> ("error out"=w718:errorcluster)  [unwired: 2 in, 2 out]
                      n179 = call <vilib>:"H5Sclose.vi"("error in (no error)"=w718, "space in"=w717) -> ("error out"=w712:errorcluster)  [unwired: 9 in]
                    }
                  }
                  n180 = call <vilib>:"H5Fclose.vi"("error in (no error)"=w664, "ref"=w663) -> ()  [unwired: 9 in, 1 out]
                }
              }
            }
          }
        }
      }
    }
  }
  "count out" <- w3
